vi "Adapt To Type.vi"(7 "Type and Defaults":variant, 8 "error in (no error)":errorcluster, 10 "Variant in":variant, 11 "Deserializer in":refnum<class "JSON Deserializer.lvclass">) -> (0 "error out":errorcluster, 2 "Variant out":variant, 3 "Deserializer out":refnum<class "JSON Deserializer.lvclass">)   [LabVIEW 2020, in "JKI JSON Serialization.lvlib" / "JSON Deserializer.lvclass"]
doc: "Adapts <b>Variant in</b> previously unflattened from a JSON formatted string to match the type of <b>Type and Defaults</b>. For any cluster element in Type and Defaults, the value of the element in Type and Default is used if element with the same name is not present in Variant in."
uses:
  JSON Deserializer.lvclass
  JSON Deserializer.lvclass/JSON Deserializer.ctl
  Library/Waveform Cluster.ctl
  Library/Empty Cluster.vi
  Library/Null Value.vi
  <userlib>/_OpenG.lib/lvdata/lvdata.llb/Get Collection Subtype__ogtk.vi
  <userlib>/_OpenG.lib/lvdata/lvdata.llb/openg_variant.lvlib
  JKI JSON Serialization.lvlib
  <vilib>/Utility/Data Type/NI_Data Type.lvlib
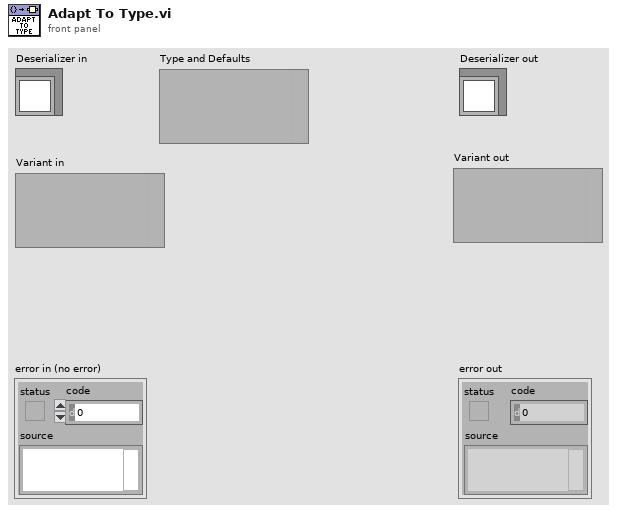
[diagram p1: front panel]
types:
  T1 = typedef "NI_Data Type.lvlib/Data Type.ctl" = enum8{"Invalid Type", "Void", "I8", "I16", "I32", "I64", "U8", "U16", "U32", "U64", "Single Float", "Double Float", "Extended Float", "Single Complex", "Double Complex", "Extended Complex", "Enum U8", "Enum U16", "Enum U32", "Enum U64", "Single Float With Unit", "Double Float With Unit", "Extended Float With Unit", "Single Complex with Unit", "Double Complex with Unit", "Extended Complex with Unit", "Boolean", "String", "Path", "Picture", "Tag", "Array", "Cluster", "Variant", "LV Variant", "Waveform", "Timestamp", "Digital Waveform", "Digital Data", "ExpressData", "Refnum", "External Data", "VI", "Poly VI", "LabVIEW Class Instance", "Fixed Point", "Set Collection", "Map Collection"}
  T2 = typedef "JKI JSON Serialization.lvlib/Waveform Cluster.ctl" = cluster{"t0":timestamp, "dt":dbl, "y":dbl[]}
  T3 = typedef "NI_Data Type.lvlib/Memory Info.ctl" = cluster{"Type":T4, "Size":u32}
  T4 = typedef "NI_Data Type.lvlib/Memory Type.ctl" = enum16{"Variable", "Fixed", "Bounded"}
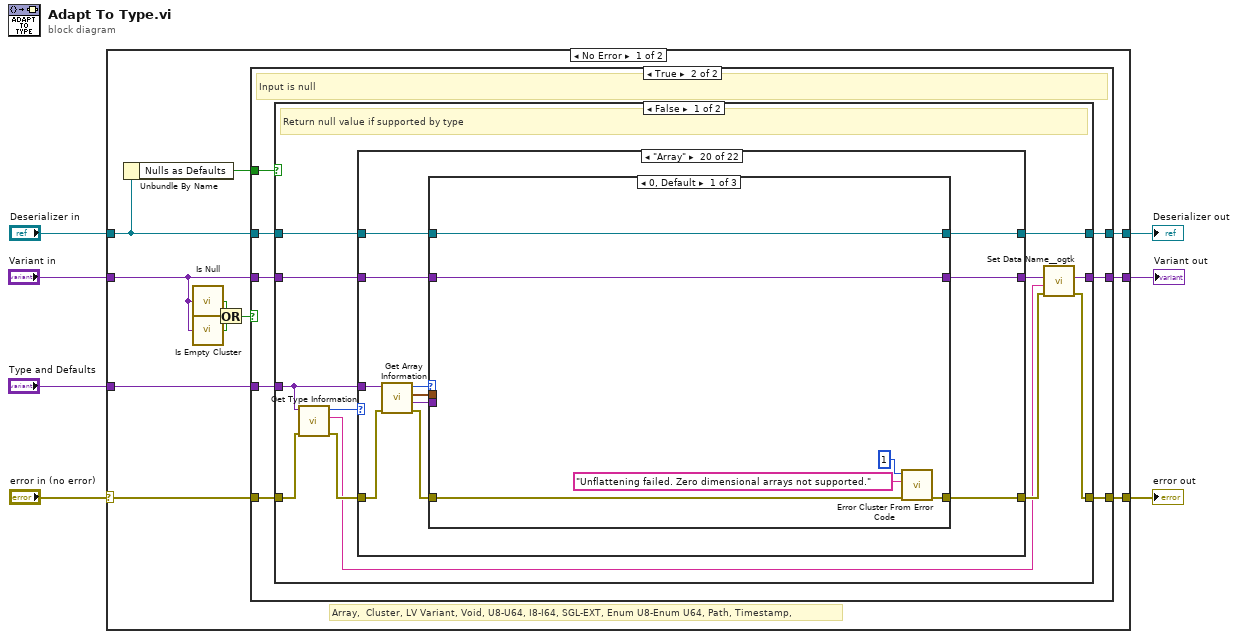
[diagram p0: block diagram]
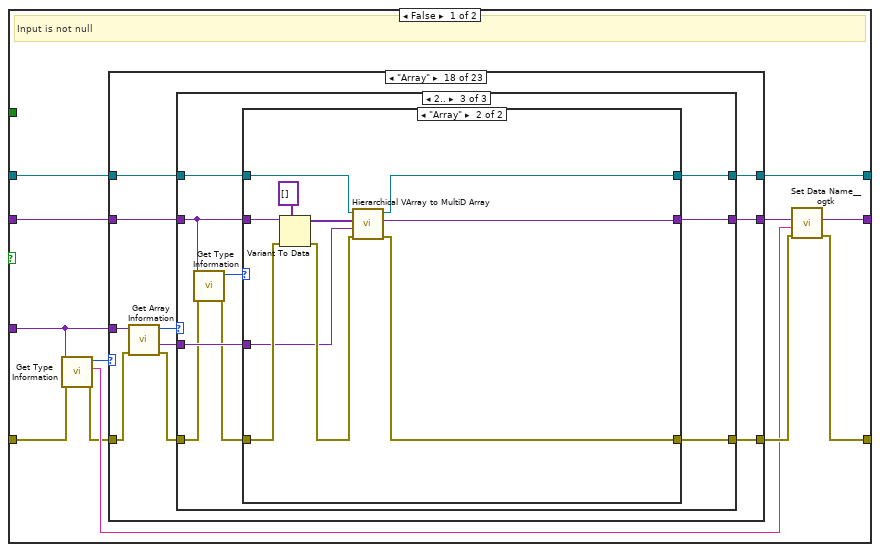
[diagram p2: hidden frame]
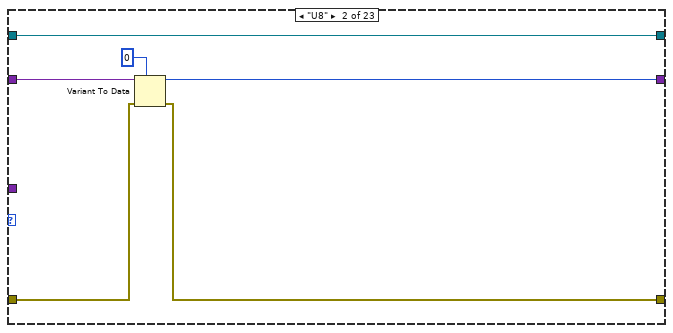
[diagram p4: hidden frame]
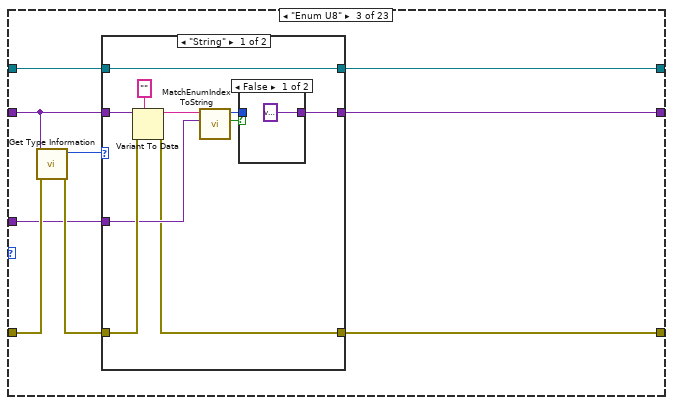
[diagram p5: hidden frame]
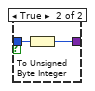
[diagram p6: hidden frame]
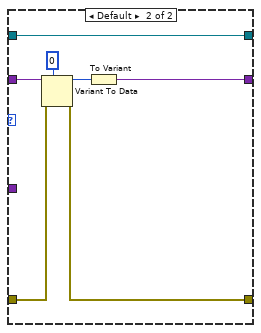
[diagram p7: hidden frame]
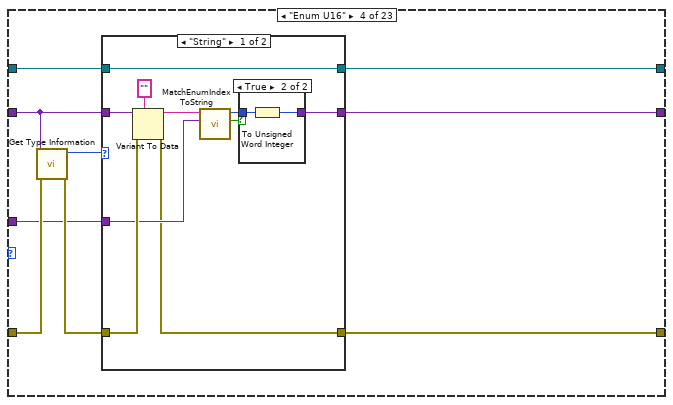
[diagram p8: hidden frame]
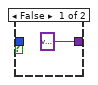
[diagram p9: hidden frame]
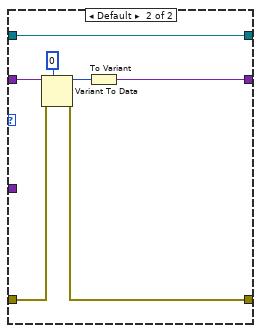
[diagram p10: hidden frame]
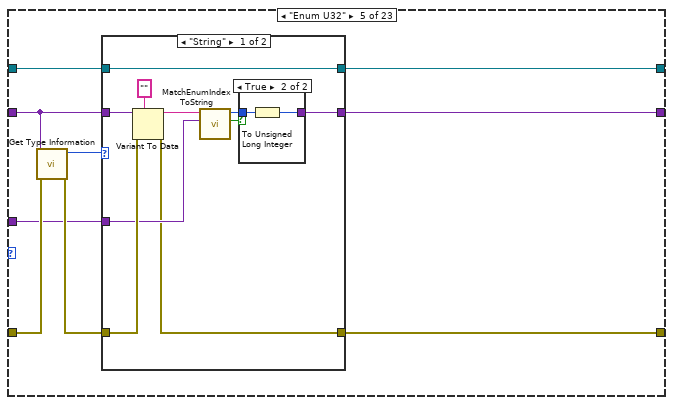
[diagram p11: hidden frame]
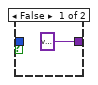
[diagram p12: hidden frame]
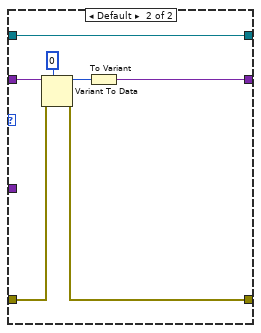
[diagram p13: hidden frame]
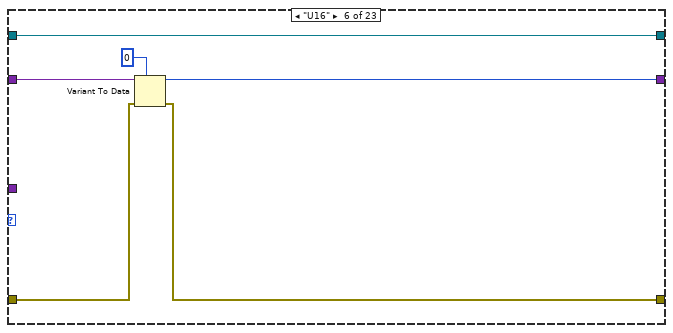
[diagram p14: hidden frame]
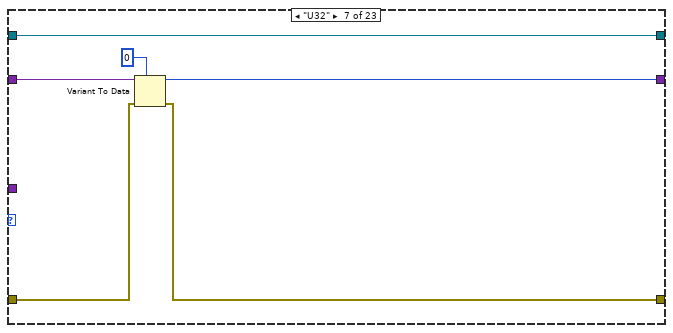
[diagram p15: hidden frame]
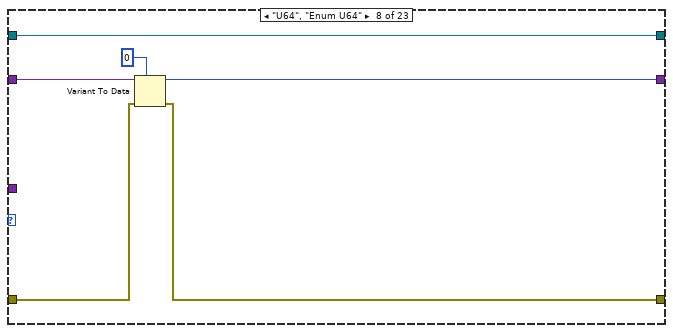
[diagram p16: hidden frame]
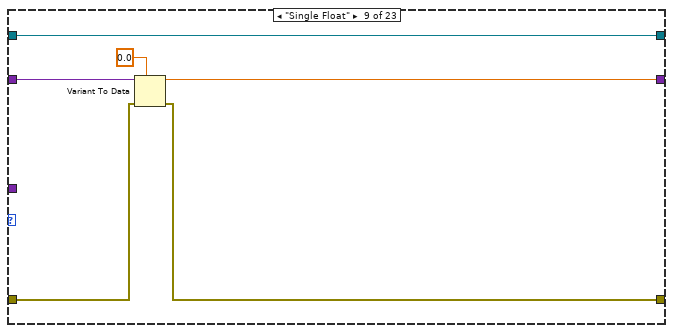
[diagram p17: hidden frame]
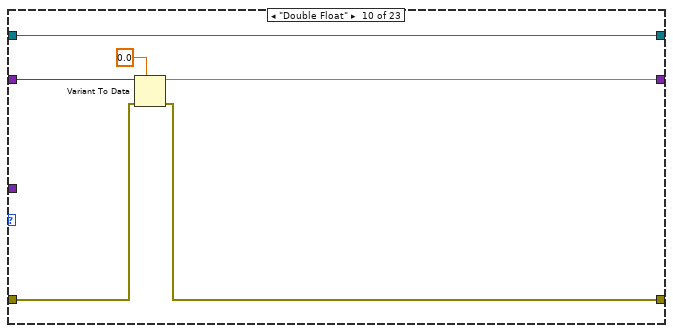
[diagram p18: hidden frame]
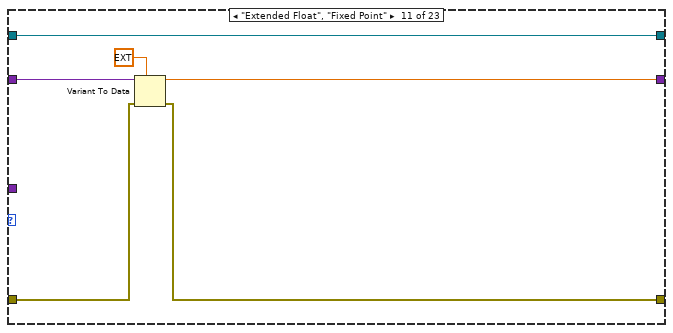
[diagram p19: hidden frame]
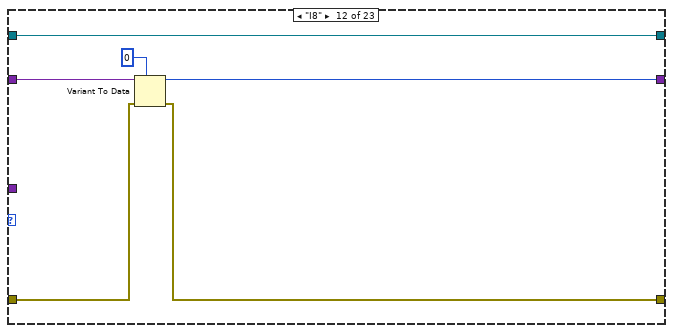
[diagram p20: hidden frame]
diagram:
  n1 = case shown="No Error" "error in (no error)" {
    selector: "error in (no error)" -> [w17 w626]
    tunnel: "Deserializer in" -> [w13 w627]
    tunnel: "Variant in" -> [w11 _]
    tunnel: [w14 w626] -> w4
    tunnel: "Type and Defaults" -> [w16 w625]
    tunnel: [w18 w627] -> w2
    tunnel: [w15 w625] -> w1
    frame No Error {
      # "Array,  Cluster, LV Variant, Void, U8-U64, I8-I64, SGL-EXT, Enum U8-Enum U64, Path, Timestamp,"
      n2 = Unbundle By Name(w13) -> ("Nulls as Defaults"=w12:bool)
      n3 = call "Is Null.vi"("Deserialized JSON Data"=w11) -> ("Null?"=w10:bool)
      n4 = call "Is Empty Cluster.vi"("Deserialized JSON Data"=w11) -> ("Empty Cluster?"=w9:bool)
      n5 = Or(x=w10, y=w9) -> (x .or. y?=w8:bool)
      n6 = case shown="True" w8 {
        tunnel: w13 -> [w20 w486]
        tunnel: [w19 w485] -> w18
        tunnel: w17 -> [w29 w483]
        tunnel: w16 -> [w28 w487]
        tunnel: [w26 w488] -> w15
        tunnel: [w25 w482] -> w14
        tunnel: w11 -> [w21 w484]
        tunnel: w12 -> [_ w481]
        frame False {
          # "Input is not null"
          n7 = call <vilib>:"Get Type Information.vi"("error in (no error)"=w29, "variant"=w28) -> ("error out"=w22:errorcluster, "name"=w23:string, "type"=w30:T1)  [unwired: 5 in, 2 out]
          n8 = case shown="\"Array\"" w30 {
            tunnel: [w32 w36 w46 w75 w104 w129 w135 w141 w147 w153 w159 w165 w171 w177 w183 w192 w195 w208 w289 w315 w345 w428 w478] -> w24
            tunnel: w22 -> [w32 w37 w44 w73 w102 w130 w136 w142 w148 w154 w160 w166 w172 w178 w184 w189 w199 w210 w306 w332 w344 w427 w478]
            tunnel: w20 -> [w33 w39 w42 w71 w100 w132 w138 w144 w150 w156 w162 w168 w174 w180 w186 w193 w201 w207 w305 w331 w349 w432 w480]
            tunnel: [w33 w39 w41 w70 w99 w132 w138 w144 w150 w156 w162 w168 w174 w180 w186 w193 w201 w205 w304 w330 w348 w431 w480] -> w19
            tunnel: w28 -> [_ _ w40 w69 w98 _ _ _ _ _ _ _ _ _ _ _ _ w211 w307 w333 w347 w430 _]
            tunnel: w21 -> [w31 w38 w47 w76 w105 w131 w137 w143 w149 w155 w161 w167 w173 w179 w185 w190 w200 w202 w302 w328 w342 w425 w479]
            tunnel: [w31 w34 w48 w77 w106 w127 w133 w139 w145 w151 w157 w163 w169 w175 w181 w191 w194 w204 w291 w317 w346 w429 w477] -> w27
            frame "Void", Default {
            }
            frame "U8" {
              n9 = Variant To Data(error in=w37, type=u8 0, Variant=w38) -> (data=w34:u8, error out=w36:errorcluster)
            }
            frame "Enum U8" {
              n10 = call <vilib>:"Get Type Information.vi"("error in (no error)"=w44, "variant"=w47) -> ("error out"=w43:errorcluster, "type"=w45:T1)  [unwired: 5 in, 3 out]
              n11 = case shown="\"String\"" w45 {
                tunnel: [w52 w62] -> w48
                tunnel: w47 -> [w58 w66]
                tunnel: w43 -> [w56 w65]
                tunnel: [w49 w64] -> w46
                tunnel: w42 -> [w50 w63]
                tunnel: [w50 w63] -> w41
                tunnel: w40 -> [w54 _]
                frame "String" {
                  n12 = Variant To Data(error in=w56, type="", Variant=w58) -> (data=w55:string, error out=w49:errorcluster)
                  n13 = call "MatchEnumIndexToString.vi"("Enum Variant"=w54, "String"=w55) -> ("found"=w51:bool, "index"=w53:i32)  [unwired: 8 in]
                  n14 = case shown="False" w51 {
                    tunnel: w53 -> [_ w61]
                    tunnel: [variant ("Type and Defaults") w60] -> w52
                    frame False {
                    }
                    frame True {
                      n15 = To Unsigned Byte Integer(number=w61) -> (unsigned 8bit integer=w60:u8)
                    }
                  }
                }
                frame Default {
                  n16 = Variant To Data(error in=w65, type=u8 0, Variant=w66) -> (data=w67:u8, error out=w64:errorcluster)
                  n17 = To Variant(anything=w67) -> (Variant=w62:variant)
                }
              }
            }
            frame "Enum U16" {
              n18 = call <vilib>:"Get Type Information.vi"("error in (no error)"=w73, "variant"=w76) -> ("error out"=w72:errorcluster, "type"=w74:T1)  [unwired: 5 in, 3 out]
              n19 = case shown="\"String\"" w74 {
                tunnel: [w81 w91] -> w77
                tunnel: w76 -> [w87 w95]
                tunnel: w72 -> [w85 w94]
                tunnel: [w78 w93] -> w75
                tunnel: w71 -> [w79 w92]
                tunnel: [w79 w92] -> w70
                tunnel: w69 -> [w83 _]
                frame "String" {
                  n20 = Variant To Data(error in=w85, type="", Variant=w87) -> (data=w84:string, error out=w78:errorcluster)
                  n21 = call "MatchEnumIndexToString.vi"("Enum Variant"=w83, "String"=w84) -> ("found"=w80:bool, "index"=w82:i32)  [unwired: 8 in]
                  n22 = case shown="True" w80 {
                    tunnel: w82 -> [_ w90]
                    tunnel: [variant ("Type and Defaults") w89] -> w81
                    frame False {
                    }
                    frame True {
                      n23 = To Unsigned Word Integer(number=w90) -> (unsigned 16bit integer=w89:u16)
                    }
                  }
                }
                frame Default {
                  n24 = Variant To Data(error in=w94, type=u16 0, Variant=w95) -> (data=w96:u16, error out=w93:errorcluster)
                  n25 = To Variant(anything=w96) -> (Variant=w91:variant)
                }
              }
            }
            frame "Enum U32" {
              n26 = call <vilib>:"Get Type Information.vi"("error in (no error)"=w102, "variant"=w105) -> ("error out"=w101:errorcluster, "type"=w103:T1)  [unwired: 5 in, 3 out]
              n27 = case shown="\"String\"" w103 {
                tunnel: [w110 w120] -> w106
                tunnel: w105 -> [w116 w124]
                tunnel: w101 -> [w114 w123]
                tunnel: [w107 w122] -> w104
                tunnel: w100 -> [w108 w121]
                tunnel: [w108 w121] -> w99
                tunnel: w98 -> [w112 _]
                frame "String" {
                  n28 = Variant To Data(error in=w114, type="", Variant=w116) -> (data=w113:string, error out=w107:errorcluster)
                  n29 = call "MatchEnumIndexToString.vi"("Enum Variant"=w112, "String"=w113) -> ("found"=w109:bool, "index"=w111:i32)  [unwired: 8 in]
                  n30 = case shown="True" w109 {
                    tunnel: w111 -> [_ w119]
                    tunnel: [variant ("Type and Defaults") w118] -> w110
                    frame False {
                    }
                    frame True {
                      n31 = To Unsigned Long Integer(number=w119) -> (unsigned 32bit integer=w118:u32)
                    }
                  }
                }
                frame Default {
                  n32 = Variant To Data(error in=w123, type=u32 0, Variant=w124) -> (data=w125:u32, error out=w122:errorcluster)
                  n33 = To Variant(anything=w125) -> (Variant=w120:variant)
                }
              }
            }
            frame "U16" {
              n34 = Variant To Data(error in=w130, type=u16 0, Variant=w131) -> (data=w127:u16, error out=w129:errorcluster)
            }
            frame "U32" {
              n35 = Variant To Data(error in=w136, type=u32 0, Variant=w137) -> (data=w133:u32, error out=w135:errorcluster)
            }
            frame "U64", "Enum U64" {
              n36 = Variant To Data(error in=w142, type=u64 0, Variant=w143) -> (data=w139:u64, error out=w141:errorcluster)
            }
            frame "Single Float" {
              n37 = Variant To Data(error in=w148, type=sgl 0.0, Variant=w149) -> (data=w145:sgl, error out=w147:errorcluster)
            }
            frame "Double Float" {
              n38 = Variant To Data(error in=w154, type=0.0, Variant=w155) -> (data=w151:dbl, error out=w153:errorcluster)
            }
            frame "Extended Float", "Fixed Point" {
              n39 = Variant To Data(error in=w160, type=ext 0.0, Variant=w161) -> (data=w157:ext, error out=w159:errorcluster)
            }
            frame "I8" {
              n40 = Variant To Data(error in=w166, type=i8 0, Variant=w167) -> (data=w163:i8, error out=w165:errorcluster)
            }
            frame "I16" {
              n41 = Variant To Data(error in=w172, type=i16 0, Variant=w173) -> (data=w169:i16, error out=w171:errorcluster)
            }
            frame "I32" {
              n42 = Variant To Data(error in=w178, type=0, Variant=w179) -> (data=w175:i32, error out=w177:errorcluster)
            }
            frame "I64" {
              n43 = Variant To Data(error in=w184, type=i64 0, Variant=w185) -> (data=w181:i64, error out=w183:errorcluster)
            }
            frame "Path" {
              n44 = Variant To Data(error in=w189, type="", Variant=w190) -> (data=w187:string, error out=w192:errorcluster)
              n45 = String To Path(string=w187) -> (path=w191:path)
            }
            frame "Timestamp" {
              n46 = Variant To Data(error in=w199, type="", Variant=w200) -> (data=w197:string, error out=w196:errorcluster)
              n47 = call "ISO String To Timestamp.vi"("error in (no error)"=w196, "ISO Timestamp String"=w197) -> ("error out"=w195:errorcluster, "Time Stamp"=w194:timestamp)  [unwired: 8 in]
            }
            frame "Array" {
              n48 = call <vilib>:"Get Array Information.vi"("error in (no error)"=w210, "variant"=w211) -> ("error out"=w209:errorcluster, "array element data type"=w206:variant, "number of dimensions"=w203:i32)  [unwired: 6 in, 1 out]
              n49 = case shown="2.." w203 {
                tunnel: w209 -> [w214 w221 w270]
                tunnel: w202 -> [w216 w219 w268]
                tunnel: [w215 w226 w275] -> w208
                tunnel: w207 -> [w217 w225 w274]
                tunnel: w206 -> [_ w224 w273]
                tunnel: [w217 w223 w272] -> w205
                tunnel: [w216 w222 w271] -> w204
                frame 0, Default {
                  n50 = call <vilib>:"Error Cluster From Error Code.vi"("error in (no error)"=w214, "error message (\"\")"="Unflattening failed. Zero dimensional arrays not supported." ("error message (\"\")"), "error code (0)"=1) -> ("error out"=w215:errorcluster)  [unwired: 6 in]
                }
                frame 1 {
                  n51 = call <vilib>:"Get Type Information.vi"("error in (no error)"=w221, "variant"=w219) -> ("error out"=w220:errorcluster, "type"=w218:T1)  [unwired: 5 in, 3 out]
                  n52 = case shown="Default" w218 {
                    tunnel: [w227 w232 w249] -> w226
                    tunnel: w225 -> [w229 w238 w259]
                    tunnel: w224 -> [w228 w231 w258]
                    tunnel: [w229 w237 w257] -> w223
                    tunnel: [w228 w234 w251] -> w222
                    tunnel: w220 -> [w227 w236 w254]
                    tunnel: w219 -> [_ w235 w256]
                    frame Default {
                    }
                    frame "Array" {
                      # "Fix GitHub Issue 28\nArray of Variants\nto Variant Array"
                      n53 = Variant To Data(error in=w236, type=variant[] [], Variant=w235) -> (data=w240:variant[], error out=w239:errorcluster)
                      n54 = for {
                        tunnel: w240 -> [w247] mode=indexing
                        shift-right: [w245] -> w233
                        shift-left: w239 -> [w246]
                        shift-right: [w243] -> w237
                        shift-left: w238 -> [w248]
                        tunnel: w231 -> [w244]
                        tunnel: [w242] -> w230 mode=indexing
                        n55 = call-dynamic "Adapt To Type.vi"("Type and Defaults"=w244, "error in (no error)"=w246, "Variant in"=w247, "Deserializer in"=w248) -> ("error out"=w245:errorcluster, "Variant out"=w242:variant, "Deserializer out"=w243:refnum<class "JSON Deserializer.lvclass">)  [unwired: 5 in]
                      }
                      n56 = call <userlib>:"Array of VData to VArray__ogtk.vi"("error in (no error)"=w233, "Element Type (when empty)"=w231, "1D Array of VData"=w230) -> ("error out"=w232:errorcluster, "VArray"=w234:variant)  [unwired: 7 in]
                    }
                    frame "Cluster" {
                      # "Fix GitHub Issue 29\nArray of Variants\nto Variant Cluster"
                      n57 = call <userlib>:"Cluster to Array of VData__ogtk.vi"("error in (no error)"=w254, "Cluster"=w256) -> ("error out"=w255:errorcluster, "Array of VData"=w253:variant[])  [unwired: 8 in]
                      n58 = for {
                        tunnel: w253 -> [w265] mode=indexing
                        shift-right: [w263] -> w250
                        shift-left: w255 -> [w264]
                        shift-right: [w261] -> w257
                        shift-left: w259 -> [w266]
                        tunnel: w258 -> [w262]
                        tunnel: [w260] -> w252 mode=indexing
                        n59 = call-dynamic "Adapt To Type.vi"("Type and Defaults"=w262, "error in (no error)"=w264, "Variant in"=w265, "Deserializer in"=w266) -> ("error out"=w263:errorcluster, "Variant out"=w260:variant, "Deserializer out"=w261:refnum<class "JSON Deserializer.lvclass">)  [unwired: 5 in]
                      }
                      n60 = call <userlib>:"Array of VData to VCluster__ogtk.vi"("error in (no error)"=w250, "Array"=w252) -> ("error out"=w249:errorcluster, "VCluster"=w251:variant)  [unwired: 8 in]
                    }
                  }
                }
                frame 2.. {
                  n61 = call <vilib>:"Get Type Information.vi"("error in (no error)"=w270, "variant"=w268) -> ("error out"=w269:errorcluster, "type"=w267:T1)  [unwired: 5 in, 3 out]
                  n62 = case shown="\"Array\"" w267 {
                    tunnel: [w276 w283] -> w275
                    tunnel: w274 -> [w278 w280]
                    tunnel: w273 -> [w277 w281]
                    tunnel: [w278 w279] -> w272
                    tunnel: [w277 w282] -> w271
                    tunnel: w269 -> [w276 w287]
                    tunnel: w268 -> [_ w286]
                    frame Default {
                    }
                    frame "Array" {
                      n63 = Variant To Data(error in=w287, type=variant[] [], Variant=w286) -> (data=w285:variant[], error out=w284:errorcluster)
                      n64 = call "Hierarchical VArray to MultiD Array.vi"("error in (no error)"=w284, "Element Type"=w281, "Hierarchical Array"=w285, "Deserializer in"=w280) -> ("error out"=w283:errorcluster, "MultiD Array"=w282:variant, "Deserializer out"=w279:refnum<class "JSON Deserializer.lvclass">)  [unwired: 5 in]
                    }
                  }
                }
              }
            }
            frame "Map Collection" {
              n65 = call <userlib>:"Map to VArray of Clusters__ogtk.vi"("error in"=w306, "Map"=w307) -> ("error out"=w294:errorcluster, "Array of Clusters (key-value)"=w295:variant)  [unwired: 8 in]
              n66 = Variant To Data(error in=w294, type=variant[] [], Variant=w295) -> (data=w293:variant[])  [unwired: 1 out]
              n67 = Index Array(array=w293) -> (element=w292:variant)  [unwired: 1 in]
              n68 = Variant To Data(type=variant[] [], Variant=w302) -> (data=w300:variant[], error out=w299:errorcluster)  [unwired: 1 in]
              n69 = for {
                tunnel: w300 -> [w313] mode=indexing
                shift-right: [w311] -> w298
                shift-left: w299 -> [w312]
                shift-right: [w309] -> w304
                shift-left: w305 -> [w314]
                tunnel: w292 -> [w310]
                tunnel: [w308] -> w297 mode=indexing
                n70 = call-dynamic "Adapt To Type.vi"("Type and Defaults"=w310, "error in (no error)"=w312, "Variant in"=w313, "Deserializer in"=w314) -> ("error out"=w311:errorcluster, "Variant out"=w308:variant, "Deserializer out"=w309:refnum<class "JSON Deserializer.lvclass">)  [unwired: 5 in]
              }
              n71 = call <userlib>:"Array of VData to VArray__ogtk.vi"("error in (no error)"=w298, "Element Type (when empty)"=w292, "1D Array of VData"=w297) -> ("error out"=w290:errorcluster, "VArray"=w303:variant)  [unwired: 7 in]
              n72 = call <userlib>:"Array of Clusters to VMap__ogtk.vi"("error in"=w290, "Array of Clusters (key-value)"=w303) -> ("error out"=w289:errorcluster, "Map"=w291:variant)  [unwired: 8 in]
            }
            frame "Set Collection" {
              n73 = call <userlib>:"Set to VArray__ogtk.vi"("error in"=w332, "Set"=w333) -> ("error out"=w320:errorcluster, "Array"=w321:variant)  [unwired: 8 in]
              n74 = Variant To Data(error in=w320, type=variant[] [], Variant=w321) -> (data=w319:variant[])  [unwired: 1 out]
              n75 = Index Array(array=w319) -> (element=w318:variant)  [unwired: 1 in]
              n76 = Variant To Data(type=variant[] [], Variant=w328) -> (data=w326:variant[], error out=w325:errorcluster)  [unwired: 1 in]
              n77 = for {
                tunnel: w326 -> [w339] mode=indexing
                shift-right: [w337] -> w324
                shift-left: w325 -> [w338]
                shift-right: [w335] -> w330
                shift-left: w331 -> [w340]
                tunnel: w318 -> [w336]
                tunnel: [w334] -> w323 mode=indexing
                n78 = call-dynamic "Adapt To Type.vi"("Type and Defaults"=w336, "error in (no error)"=w338, "Variant in"=w339, "Deserializer in"=w340) -> ("error out"=w337:errorcluster, "Variant out"=w334:variant, "Deserializer out"=w335:refnum<class "JSON Deserializer.lvclass">)  [unwired: 5 in]
              }
              n79 = call <userlib>:"Array of VData to VArray__ogtk.vi"("error in (no error)"=w324, "Element Type (when empty)"=w318, "1D Array of VData"=w323) -> ("error out"=w316:errorcluster, "VArray"=w329:variant)  [unwired: 7 in]
              n80 = call <userlib>:"Array to Set__ogtk.vi"("error in"=w316, "Array"=w329) -> ("error out"=w315:errorcluster, "Set"=w317:variant)  [unwired: 8 in]
            }
            frame "Cluster" {
              n81 = call <vilib>:"Get Type Information.vi"("error in (no error)"=w344, "variant"=w342) -> ("error out"=w343:errorcluster, "type"=w341:T1)  [unwired: 5 in, 3 out]
              n82 = case shown="\"Array\"" w341 {
                tunnel: w349 -> [w355 w358 w364 w396]
                tunnel: [w355 w358 w363 w395] -> w348
                tunnel: w347 -> [w354 w357 w370 w394]
                tunnel: [w354 w357 w361 w386] -> w346
                tunnel: [w353 w356 w359 w383] -> w345
                tunnel: w343 -> [w352 w356 w369 w382]
                tunnel: w342 -> [_ _ w371 w381]
                frame "Invalid Type", Default {
                  n83 = call <vilib>:"Error Cluster From Error Code.vi"("error in (no error)"=w352, "error message (\"\")"="Cannot deserialize the input type into a cluster." ("error message (\"\")"), "error code (0)"=1) -> ("error out"=w353:errorcluster)  [unwired: 6 in]
                }
                frame "Void" {
                  # "Empty input object, use default values"
                }
                frame "Array" {
                  n84 = call <userlib>:"Cluster to Array of VData__ogtk.vi"("error in (no error)"=w369, "Cluster"=w370) -> ("error out"=w368:errorcluster, "Array of VData"=w367:variant[])  [unwired: 8 in]
                  n85 = call <userlib>:"Array to Array of VData__ogtk.vi"("error in (no error)"=w368, "MultiD Array"=w371) -> ("error out"=w365:errorcluster, "1D Array of Variants"=w366:variant[])  [unwired: 8 in]
                  n86 = for {
                    tunnel: w367 -> [w376] mode=indexing
                    tunnel: w366 -> [w379]
                    shift-right: [w374] -> w360
                    shift-left: w365 -> [w375]
                    shift-right: [w373] -> w363
                    shift-left: w364 -> [w380]
                    tunnel: [w372] -> w362 mode=indexing
                    i -> [w378]
                    n87 = Index Array(array=w379, index=w378) -> (element=w377:variant)
                    n88 = call-dynamic "Adapt To Type.vi"("Type and Defaults"=w376, "error in (no error)"=w375, "Variant in"=w377, "Deserializer in"=w380) -> ("error out"=w374:errorcluster, "Variant out"=w372:variant, "Deserializer out"=w373:refnum<class "JSON Deserializer.lvclass">)  [unwired: 5 in]
                  }
                  n89 = call <userlib>:"Array of VData to VCluster__ogtk.vi"("error in (no error)"=w360, "Array"=w362) -> ("error out"=w359:errorcluster, "VCluster"=w361:variant)  [unwired: 8 in]
                }
                frame "Cluster" {
                  n90 = call <userlib>:"Cluster to Array of VData__ogtk.vi"("error in (no error)"=w382, "Cluster"=w394) -> ("error out"=w392:errorcluster, "Array of VData"=w393:variant[])  [unwired: 8 in]
                  n91 = call <userlib>:"Cluster to Array of VData__ogtk.vi"("error in (no error)"=w392, "Cluster"=w381) -> ("error out"=w388:errorcluster, "Array of VData"=w391:variant[])  [unwired: 8 in]
                  n92 = for {
                    tunnel: w391 -> [w398] mode=indexing
                    shift-right: [w399] -> w387
                    shift-left: w388 -> [w400]
                    tunnel: [w398] -> w390 mode=indexing
                    tunnel: [w397] -> w389 mode=indexing
                    n93 = call <vilib>:"Get Type Information.vi"("error in (no error)"=w400, "variant"=w398) -> ("error out"=w399:errorcluster, "name"=w397:string)  [unwired: 5 in, 3 out]
                  }
                  n94 = for {
                    shift-right: [w410] -> w384
                    shift-left: w387 -> [w405]
                    shift-right: [w409] -> w395
                    shift-left: w396 -> [w411]
                    tunnel: w393 -> [w402] mode=indexing
                    tunnel: [w408] -> w385 mode=indexing
                    tunnel: w390 -> [w403]
                    tunnel: w389 -> [w407]
                    n95 = call <vilib>:"Get Type Information.vi"("error in (no error)"=w405, "variant"=w402) -> ("error out"=w404:errorcluster, "name"=w406:string)  [unwired: 5 in, 3 out]
                    n96 = Search 1D Array(1D array=w407, element=w406) -> (index of element=w401:i32)  [unwired: 1 in]
                    n97 = case shown="0.." w401 {
                      selector: w401 -> [_ w415]
                      tunnel: w411 -> [w414 w423]
                      tunnel: [w412 w422] -> w410
                      tunnel: [w414 w421] -> w409
                      tunnel: [w413 w420] -> w408
                      tunnel: w404 -> [w412 w419]
                      tunnel: w403 -> [_ w418]
                      tunnel: w402 -> [w413 w416]
                      frame ..-1 {
                        # "Element not found"
                      }
                      frame 0.. {
                        # "Element found"
                        n98 = Index Array(array=w418, index=w415) -> (element=w417:variant)
                        n99 = call-dynamic "Adapt To Type.vi"("Type and Defaults"=w416, "error in (no error)"=w419, "Variant in"=w417, "Deserializer in"=w423) -> ("error out"=w422:errorcluster, "Variant out"=w420:variant, "Deserializer out"=w421:refnum<class "JSON Deserializer.lvclass">)  [unwired: 5 in]
                      }
                    }
                  }
                  n100 = call <userlib>:"Array of VData to VCluster__ogtk.vi"("error in (no error)"=w384, "Array"=w385) -> ("error out"=w383:errorcluster, "VCluster"=w386:variant)  [unwired: 8 in]
                }
              }
            }
            frame "Waveform" {
              n101 = call <vilib>:"Get Type Information.vi"("error in (no error)"=w427, "variant"=w425) -> ("error out"=w426:errorcluster, "type"=w424:T1)  [unwired: 5 in, 3 out]
              n102 = case shown="\"Array\"" w424 {
                tunnel: w432 -> [w438 w441 w456 w473]
                tunnel: [w438 w441 w443 w466] -> w431
                tunnel: w430 -> [w437 w440 w458 w475]
                tunnel: [w437 w440 w442 w465] -> w429
                tunnel: [w436 w439 w444 w467] -> w428
                tunnel: w426 -> [w435 w439 w457 w474]
                tunnel: w425 -> [_ _ w454 w472]
                frame "Invalid Type", Default {
                  n103 = call <vilib>:"Error Cluster From Error Code.vi"("error in (no error)"=w435, "error message (\"\")"="Cannot deserialize the input type into a waveform." ("error message (\"\")"), "error code (0)"=1) -> ("error out"=w436:errorcluster)  [unwired: 6 in]
                }
                frame "Void" {
                  # "Empty input object, use default values"
                }
                frame "Cluster" {
                  w450 = T2 {"t0"=timestamp(0 s since 1904-01-01), "dt"=1.0, "y"=[]}  # waveform
                  n104 = Variant To Data(error in=w457, type=waveform(dbl) {"t0"=timestamp(0 s since 1904-01-01), "dt"=1.0, "Y"=[]}, Variant=w458) -> (data=w449:waveform(dbl), error out=w453:errorcluster)
                  n105 = Unbundle By Name(w449) -> ("t0"=w461:timestamp, "dt"=w460:dbl, "Y"=w459:dbl[])
                  n106 = Bundle By Name(cluster=w450, "t0"=w461, "dt"=w460, "y"=w459) -> (w455:T2)
                  n107 = call-dynamic "Adapt To Type.vi"("Type and Defaults"=w455, "error in (no error)"=w453, "Variant in"=w454, "Deserializer in"=w456) -> ("error out"=w451:errorcluster, "Variant out"=w452:variant, "Deserializer out"=w443:refnum<class "JSON Deserializer.lvclass">)  [unwired: 5 in]
                  n108 = Variant To Data(error in=w451, type=w450, Variant=w452) -> (data=w448:T2, error out=w444:errorcluster)
                  n109 = Unbundle By Name(w448) -> ("t0"=w447:timestamp, "dt"=w446:dbl, "y"=w445:dbl[])
                  n110 = Bundle By Name(cluster=w449, "t0"=w447, "dt"=w446, "Y"=w445) -> (w442:waveform(dbl))
                }
                frame "Array" {
                  n111 = Variant To Data(error in=w474, type=waveform(dbl) {"t0"=timestamp(0 s since 1904-01-01), "dt"=1.0, "Y"=[]}, Variant=w475) -> (data=w468:waveform(dbl), error out=w471:errorcluster)
                  n112 = Unbundle By Name(w468) -> ("Y"=w464:dbl[])
                  n113 = call-dynamic "Adapt To Type.vi"("Type and Defaults"=w464, "error in (no error)"=w471, "Variant in"=w472, "Deserializer in"=w473) -> ("error out"=w469:errorcluster, "Variant out"=w470:variant, "Deserializer out"=w466:refnum<class "JSON Deserializer.lvclass">)  [unwired: 5 in]
                  n114 = Variant To Data(error in=w469, type=w464, Variant=w470) -> (data=w463:dbl[], error out=w467:errorcluster)
                  n115 = Bundle By Name(cluster=w468, "Y"=w463) -> (w465:waveform(dbl))
                }
              }
            }
            frame "LV Variant" {
              n116 = To Variant(anything=w479) -> (Variant=w477:variant)
            }
          }
          n117 = call <userlib>:"Set Data Name__ogtk.vi"("error in (no error)"=w24, "Data Name"=w23, "Data"=w27) -> ("error out"=w25:errorcluster, "Renamed Data"=w26:variant)  [unwired: 7 in]
        }
        frame True {
          # "Input is null"
          n118 = case shown="False" w481 {
            tunnel: [w496 w624] -> w488
            tunnel: w487 -> [w493 w624]
            tunnel: w486 -> [w500 w623]
            tunnel: [w499 w623] -> w485
            tunnel: w484 -> [w498 _]
            tunnel: w483 -> [w492 w622]
            tunnel: [w494 w622] -> w482
            frame False {
              # "Return null value if supported by type"
              n119 = call <vilib>:"Get Type Information.vi"("error in (no error)"=w492, "variant"=w493) -> ("error out"=w491:errorcluster, "name"=w489:string, "type"=w490:T1)  [unwired: 5 in, 2 out]
              n120 = case shown="\"Array\"" w490 {
                tunnel: [w502 w504 w507 w510 w513 w516 w519 w522 w525 w528 w531 w534 w537 w540 w543 w546 w549 w554 w559 w570 w598 w610] -> w495
                tunnel: w491 -> [w502 w504 w507 w510 w513 w516 w519 w522 w525 w528 w531 w534 w537 w540 w543 w546 w549 w554 w561 w572 w609 w621]
                tunnel: w500 -> [w503 w506 w509 w512 w515 w518 w521 w524 w527 w530 w533 w536 w539 w542 w545 w548 w551 w555 w562 w569 w608 w620]
                tunnel: [w503 w506 w509 w512 w515 w518 w521 w524 w527 w530 w533 w536 w539 w542 w545 w548 w551 w555 w562 w567 w608 w620] -> w499
                tunnel: w493 -> [_ _ _ _ _ _ _ _ _ _ _ _ _ _ _ _ _ _ w558 w573 w606 w618]
                tunnel: w498 -> [w501 _ _ _ _ _ _ _ _ _ _ _ _ _ _ _ _ w553 _ w564 _ _]
                tunnel: [w501 "" path "" waveform(dbl) {"t0"=timestamp(0 s since 1904-01-01), "dt"=1.0, "Y"=[]} FALSE timestamp(0 s since 1904-01-01) sgl nan nan ext nan u8 0 u16 0 u32 0 u64 0 i8 0 i16 0 0 i64 0 w552 w556 w566 w601 w613] -> w497
                frame "Void", Default {
                }
                frame "String" {
                }
                frame "Path" {
                }
                frame "Waveform" {
                }
                frame "Boolean" {
                }
                frame "Timestamp" {
                }
                frame "Single Float" {
                }
                frame "Double Float" {
                }
                frame "Extended Float", "Fixed Point" {
                }
                frame "U8", "Enum U8" {
                }
                frame "U16", "Enum U16" {
                }
                frame "U32", "Enum U32" {
                }
                frame "U64", "Enum U64" {
                }
                frame "I8" {
                }
                frame "I16" {
                }
                frame "I32" {
                }
                frame "I64" {
                }
                frame "LV Variant" {
                  n121 = To Variant(anything=w553) -> (Variant=w552:variant)
                }
                frame "Cluster" {
                  # "Get cluster default value"
                  n122 = call <vilib>:"Get Cluster Information.vi"("error in (no error)"=w561, "variant"=w558) -> ("error out"=w560:errorcluster, "cluster elements"=w557:variant[])  [unwired: 8 in]
                  n123 = call <vilib>:"Set Cluster Information.vi"("error in (no error)"=w560, "Cluster Elements"=w557, "Variant in"=w558) -> ("error out"=w559:errorcluster, "Variant out"=w556:variant)  [unwired: 7 in]
                }
                frame "Array" {
                  n124 = call <vilib>:"Get Array Information.vi"("error in (no error)"=w572, "variant"=w573) -> ("error out"=w571:errorcluster, "array element data type"=w568:variant, "array lengths"=w563:T3[], "number of dimensions"=w565:i32)  [unwired: 6 in]
                  n125 = case shown="0, Default" w565 {
                    tunnel: w571 -> [w576 w583 w596]
                    tunnel: w564 -> [w578 _ _]
                    tunnel: [w577 w580 w590] -> w570
                    tunnel: w569 -> [w579 w584 w597]
                    tunnel: w568 -> [_ w582 w595]
                    tunnel: [w579 w584 w597] -> w567
                    tunnel: [w578 w585 w592] -> w566
                    tunnel: w563 -> [_ _ w589]
                    frame 0, Default {
                      n126 = call <vilib>:"Error Cluster From Error Code.vi"("error in (no error)"=w576, "error message (\"\")"="Unflattening failed. Zero dimensional arrays not supported." ("error message (\"\")"), "error code (0)"=1) -> ("error out"=w577:errorcluster)  [unwired: 6 in]
                    }
                    frame 1 {
                      n127 = call <userlib>:"Array of VData to VArray__ogtk.vi"("error in (no error)"=w583, "Element Type (when empty)"=w582, "1D Array of VData"=variant[] []) -> ("error out"=w580:errorcluster, "VArray"=w585:variant)  [unwired: 7 in]
                    }
                    frame 2.. {
                      n128 = Array Size(array=w589) -> (size(s)=w588:i32)
                      n129 = Initialize Array(0, w588) -> (w586:i32[])
                      n130 = call <userlib>:"Array of VData to VArray__ogtk.vi"("error in (no error)"=w596, "Element Type (when empty)"=w595, "1D Array of VData"=variant[] []) -> ("error out"=w591:errorcluster, "VArray"=w593:variant)  [unwired: 7 in]
                      n131 = call <userlib>:"Reshape 1D Array__ogtk.vi"("error in (no error)"=w591, "Size(s)"=w586, "1D Array"=w593) -> ("error out"=w590:errorcluster, "Reshaped VArray"=w592:variant)  [unwired: 7 in]
                    }
                  }
                }
                frame "Map Collection" {
                  # "#todo test null map support"
                  n132 = call <userlib>:"Map to VArray of Clusters__ogtk.vi"("error in"=w609, "Map"=w606) -> ("error out"=w607:errorcluster, "Array of Clusters (key-value)"=w605:variant)  [unwired: 8 in]
                  n133 = call <vilib>:"Get Array Information.vi"("error in (no error)"=w607, "variant"=w605) -> ("error out"=w600:errorcluster, "array element data type"=w603:variant)  [unwired: 6 in, 2 out]
                  n134 = call <userlib>:"Array of VData to VArray__ogtk.vi"("error in (no error)"=w600, "Element Type (when empty)"=w603, "1D Array of VData"=variant[] []) -> ("error out"=w599:errorcluster, "VArray"=w602:variant)  [unwired: 7 in]
                  n135 = call <userlib>:"Array of Clusters to VMap__ogtk.vi"("error in"=w599, "Array of Clusters (key-value)"=w602) -> ("error out"=w598:errorcluster, "Map"=w601:variant)  [unwired: 8 in]
                }
                frame "Set Collection" {
                  # "#todo test null set support"
                  n136 = call <userlib>:"Set to VArray__ogtk.vi"("error in"=w621, "Set"=w618) -> ("error out"=w619:errorcluster, "Array"=w617:variant)  [unwired: 8 in]
                  n137 = call <vilib>:"Get Array Information.vi"("error in (no error)"=w619, "variant"=w617) -> ("error out"=w612:errorcluster, "array element data type"=w615:variant)  [unwired: 6 in, 2 out]
                  n138 = call <userlib>:"Array of VData to VArray__ogtk.vi"("error in (no error)"=w612, "Element Type (when empty)"=w615, "1D Array of VData"=variant[] []) -> ("error out"=w611:errorcluster, "VArray"=w614:variant)  [unwired: 7 in]
                  n139 = call <userlib>:"Array to Set__ogtk.vi"("error in"=w611, "Array"=w614) -> ("error out"=w610:errorcluster, "Set"=w613:variant)  [unwired: 8 in]
                }
              }
              n140 = call <userlib>:"Set Data Name__ogtk.vi"("error in (no error)"=w495, "Data Name"=w489, "Data"=w497) -> ("error out"=w494:errorcluster, "Renamed Data"=w496:variant)  [unwired: 7 in]
            }
            frame True {
              # "Return default value"
            }
          }
        }
      }
    }
    frame Error {
    }
  }
  "error out" <- w4
  "Deserializer out" <- w2
  "Variant out" <- w1
